vi "Log_ADAM_scan_table.vi"() -> ()   [LabVIEW 2010]
uses:
  ADAM Client/Sub VIs/ADAM Controls/Channel_State.ctl
  Anemometry/Anemometry Sub Vis/Globals/Constants_global.vi
  Anemometry/Anemometry Sub Vis/Globals/Preference_global.vi
  ADAM_Global.vi
  Anemometry/Anemometry Sub Vis/Globals/Meas_global.vi
panel:
  in  "Averaging time (Seconds)":dbl=60.0
  out "Current time":string
  out "Started Time":string
  in  "stop":bool
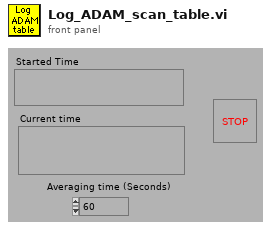
[diagram p1: front panel]
types:
  T1 = enum16{"On", "Off", "Always On", "Always Off", "Delete"}
  T2 = typedef "Channel_State.ctl" = enum16{"On", "Off", "Always On", "Always Off"}
  T3 = enum16{"Load ADAM setup from excel file", "Save ADAM setup to excel file"}
  T4 = cluster{"second":i32, "minute":i32, "hour":i32, "day of month":i32, "month":i32, "year":i32, "day of week":i32, "day of year":i32, "is DST":i32}
  T5 = typedef "Client_State_Cluster.ctl" = cluster{"Client Name":string, "Traverse level State":T6, "People to Email":string[], "Next Contact Time":dbl}
  T6 = typedef "Traverse_Level_State.ctl" = enum16{"Running", "Complete"}
  T7 = typedef "Server_Control.ctl" = cluster{"Channel Name to control":string, "Channel sharing":enum16{"Channel Unshared", "Channel Shared by Rig", "Channel Shared by Group"}, "Default Value":dbl, "Client Array":string[], "Time Stamp":timestamp, "Do Not Reset":bool}
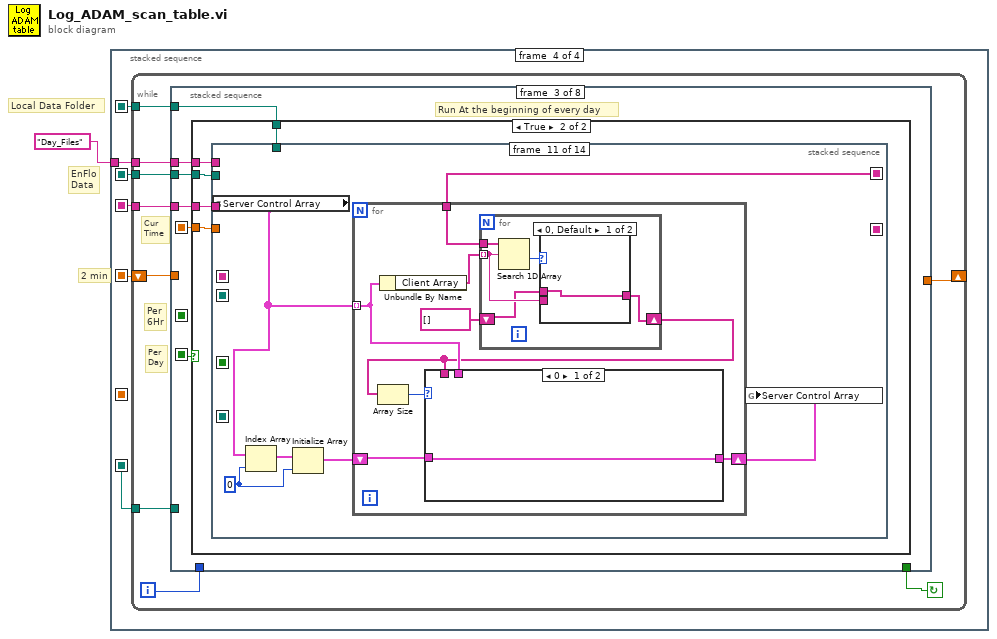
[diagram p0: block diagram]
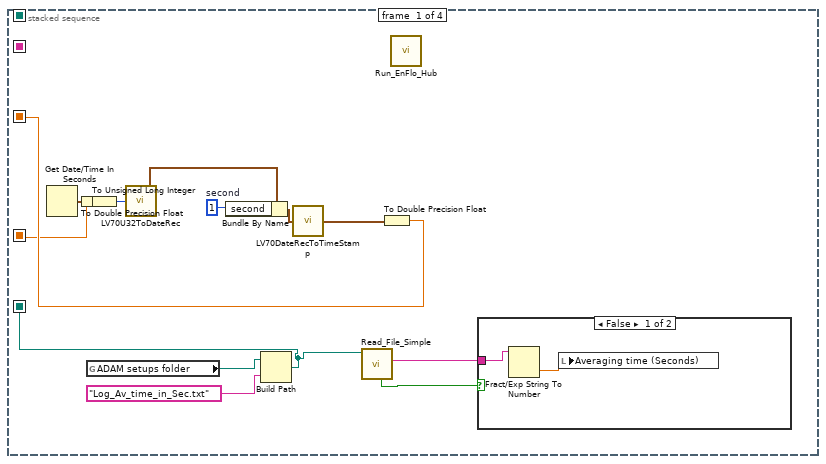
[diagram p2: hidden frame]
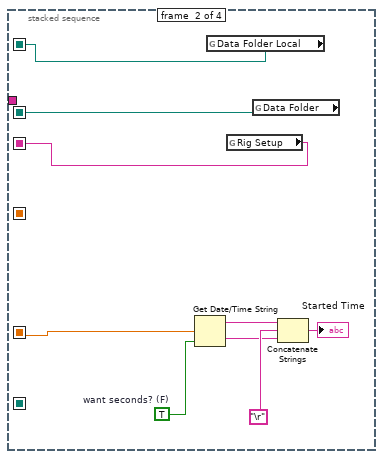
[diagram p4: hidden frame]
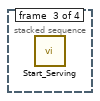
[diagram p5: hidden frame]
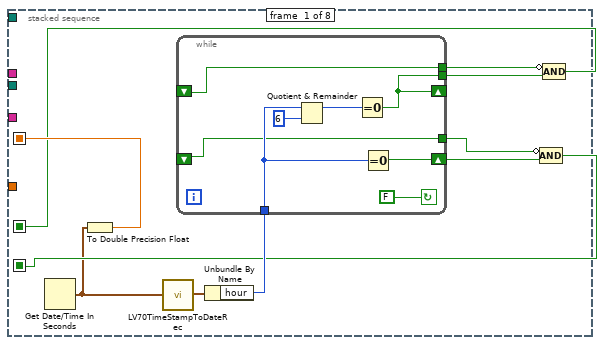
[diagram p6: hidden frame]
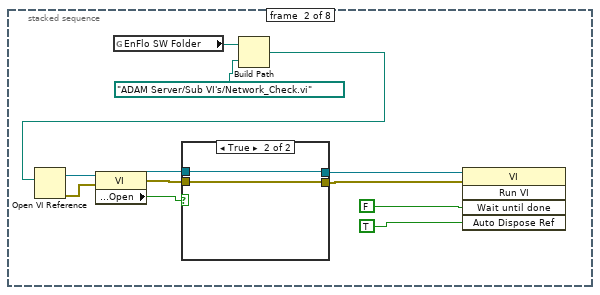
[diagram p7: hidden frame]
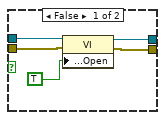
[diagram p8: hidden frame]
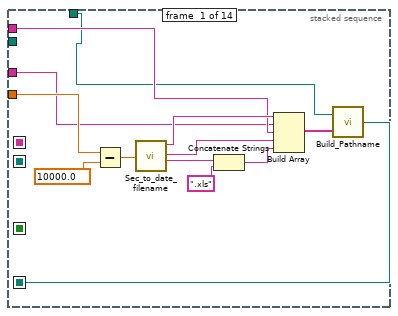
[diagram p10: hidden frame]
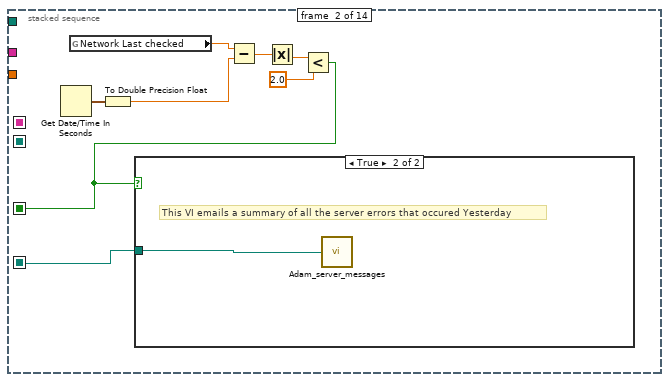
[diagram p11: hidden frame]
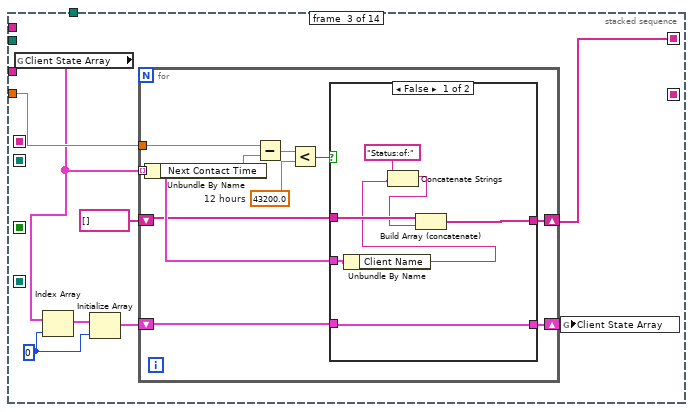
[diagram p13: hidden frame]
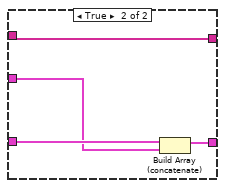
[diagram p14: hidden frame]
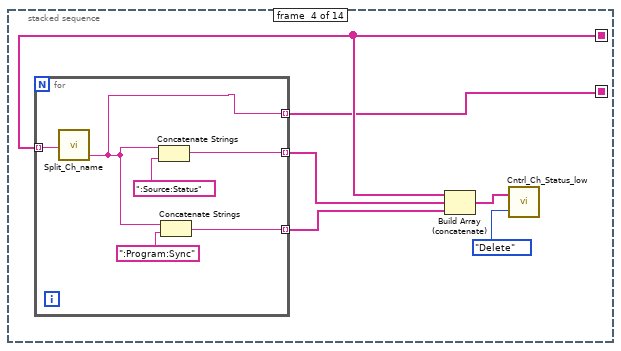
[diagram p15: hidden frame]
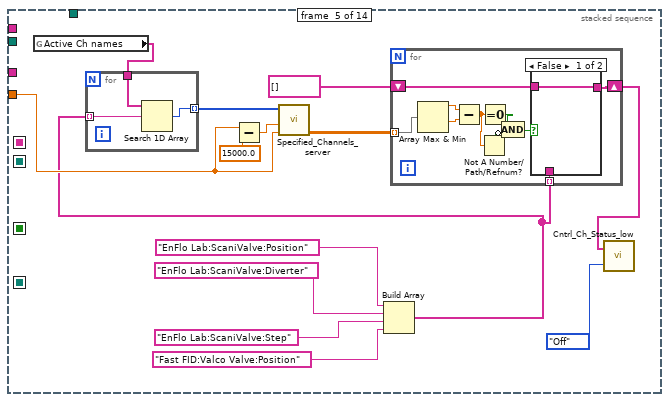
[diagram p16: hidden frame]
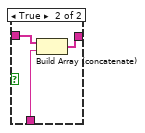
[diagram p17: hidden frame]
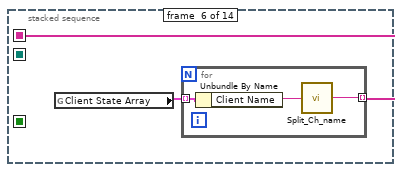
[diagram p18: hidden frame]
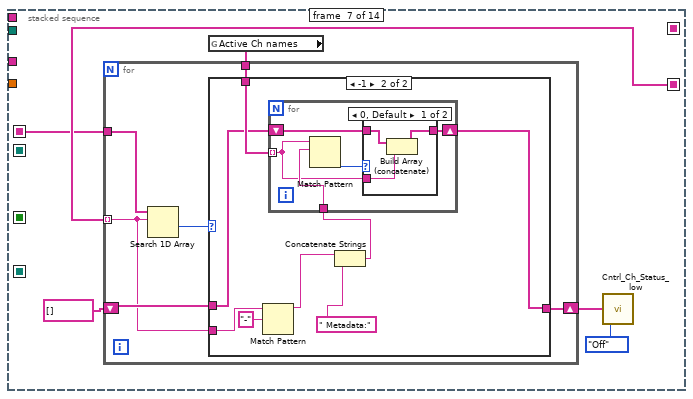
[diagram p19: hidden frame]
diagram:
  # "Local Data Folder"
  # "EnFlo\nData"
  # "2 min"
  n1 = stacked-sequence {
    seq-local: [w12 _ _ _] -> [_ _ _ w31]
    seq-local: [w11 _ _ _] -> [_ w25 _ _]
    seq-local: [_ w19 _ _] -> [_ _ _ w30]
    seq-local: [w4 _ _ _] -> [_ _ _ w28]
    seq-local: [_ w18 _ _] -> [_ _ _ w27]
    seq-local: [_ w17 _ _] -> [_ _ _ w26]
    tunnel: "Day_Files" ("Input Element") -> [_ _ _ w29]
    frame #0 {
      w14 = 1  # second
      n2 = Get Date/Time In Seconds() -> (seconds since 1Jan1904=w8:timestamp)
      n3 = To Double Precision Float(number=w8) -> (double precision float=w11:dbl)
      n4 = global read "Constants_global.vi" "ADAM setups folder"() -> (w6:path)
      n5 = To Unsigned Long Integer(number=w11) -> (unsigned 32bit integer=w10:u32)
      n6 = call <vilib>:"LV70U32ToDateRec.vi"("Time"=w10) -> ("date time rec"=w9:T4)
      n7 = Bundle By Name(cluster=w9, "second"=w14) -> (w13:T4)
      n8 = Build Path(base path=w6, name or relative path="Log_Av_time_in_Sec.txt") -> (appended path=w4:path)
      n9 = call <vilib>:"LV70DateRecToTimeStamp.vi"("date time rec"=w13) -> ("Time Stamp"=w7:timestamp)
      n10 = call "Read_File_Simple.vi"("Filename"=w4) -> ("Error?"=w2:bool, "string"=w3:string)  [unwired: 2 in, 6 out]
      n11 = To Double Precision Float(number=w7) -> (double precision float=w12:dbl)
      n12 = call "Run_EnFlo_Hub.vi"() -> ()  [unwired: 8 out]
      n13 = case shown="False" w2 {
        tunnel: w3 -> [w16 _]
        frame False {
          n14 = Fract/Exp String To Number(string=w16) -> (number=w15:dbl)  [unwired: 4 out]
          n15 = local write "Averaging time (Seconds)"(w15) -> ()
        }
        frame True {
        }
      }
    }
    frame #1 {
      w24 = TRUE  # want seconds? (F)
      n16 = Get Date/Time String(seconds (now)=w25, want seconds? (F)=w24) -> (date string=w22:string, time string=w21:string)  [unwired: 1 out]
      n17 = global read "Constants_global.vi" "Data Folder Local"() -> (w17:path)
      n18 = global read "Preference_global.vi" "Rig Setup"() -> (w18:string)
      n19 = global read "Constants_global.vi" "Data Folder"() -> (w19:path)
      n20 = Concatenate Strings(w22, "\r", w21) -> (→"Started Time":string)
    }
    frame #2 {
      n21 = call "Start_Serving.vi"() -> ()  [unwired: 1 out]
    }
    frame #3 {
      n22 = while {
        tunnel: w30 -> [w38]
        shift-left: w31 -> [w40]
        shift-right: [w39] -> _
        tunnel: w29 -> [w35]
        tunnel: w28 -> [w34]
        tunnel: w27 -> [w33]
        tunnel: w26 -> [w32]
        i -> [w37]
        stop <- w36 continue-if-true
        # "Per\n6Hr"
        # "Per\nDay"
        # "Cur\nTime"
        n23 = stacked-sequence {
          seq-local: [w42 _ _ _ _ _ _ _] -> [_ _ w83 _ _ _ _ _]
          seq-local: [w49 _ _ _ _ _ _ _] -> [_ _ w82 w342 _ w359 _ _]
          seq-local: [w45 _ _ _ _ _ _ _] -> [_ _ _ w336 _ _ _ _]
          tunnel: [_ _ _ _ _ w358 _ _] -> w39
          tunnel: w40 -> [_ _ _ _ _ w360 _ _]
          tunnel: w38 -> [_ _ w81 _ _ w367 _ _]
          tunnel: w37 -> [_ _ _ w335 _ _ _ _]
          tunnel: [_ _ _ _ _ _ _ w416] -> w36
          tunnel: w35 -> [_ _ w80 _ _ w368 _ _]
          tunnel: w34 -> [_ _ _ _ _ _ _ w415]
          tunnel: w33 -> [_ _ w79 _ _ w361 _ _]
          tunnel: w32 -> [_ _ w78 _ _ w357 _ _]
          frame #0 {
            n24 = Get Date/Time In Seconds() -> (seconds since 1Jan1904=w41:timestamp)
            n25 = To Double Precision Float(number=w41) -> (double precision float=w49:dbl)
            n26 = call <vilib>:"LV70TimeStampToDateRec.vi"("time stamp"=w41) -> ("date time rec"=w50:T4)
            n27 = Unbundle By Name(w50) -> ("hour"=w48:i32)
            n28 = while {
              tunnel: [w52] -> w43
              shift-left: _ -> [w52]
              shift-right: [w53] -> w44
              tunnel: [w55] -> w46
              tunnel: [w56] -> w47
              tunnel: w48 -> [w54]
              shift-left: _ -> [w55]
              shift-right: [w56] -> _
              stop <- FALSE continue-if-true
              n29 = Quotient & Remainder(x=w54, y=6) -> (x-y*floor(x/y)=w57:i32)  [unwired: 1 out]
              n30 = Equal To 0?(x=w57) -> (x = 0?=w56:bool)
              n31 = Equal To 0?(x=w54) -> (x = 0?=w53:bool)
            }
            n32 = Compound Arithmetic op=AND(invert w43, w44) -> (w42:bool)
            n33 = Compound Arithmetic op=AND(invert w46, w47) -> (w45:bool)
          }
          frame #1 {
            n34 = global read "Constants_global.vi" "EnFlo SW Folder"() -> (w68:path)
            n35 = Build Path(base path=w68, name or relative path=path "ADAM Server/Sub VI's/Network_Check.vi") -> (appended path=w69:path)
            n36 = Open VI Reference(vi path=w69) -> (vi reference=w65:refnum<vi>, error out=w64:errorcluster)  [unwired: 1 in, 4 out]
            n37 = property class="VI"(reference=w65, error in=w64) -> (reference out=w62:refnum<vi>, error out=w61:errorcluster, "Front Panel Window:Open"=w63:bool)
            n38 = case shown="True" w63 {
              tunnel: w62 -> [w74 w77]
              tunnel: w61 -> [w73 w76]
              tunnel: [w72 w77] -> w60
              tunnel: [w71 w76] -> w59
              frame False {
                n39 = property class="VI"(reference=w74, error in=w73, "Front Panel Window:Open"=TRUE) -> (reference out=w72:refnum<vi>, error out=w71:errorcluster)
              }
              frame True {
              }
            }
            n40 = invoke class="VI" method="Run VI"(reference=w60, error in=w59, "Wait until done"=FALSE, "Auto Dispose Ref"=TRUE) -> ()  [unwired: 1 in, 5 out]
          }
          frame #2 {
            # "Run At the beginning of every day"
            n41 = case shown="True" w83 {
              tunnel: w82 -> [_ w88]
              tunnel: w81 -> [_ w87]
              tunnel: w80 -> [_ w86]
              tunnel: w79 -> [_ w85]
              tunnel: w78 -> [_ w84]
              frame False {
              }
              frame True {
                n42 = stacked-sequence {
                  seq-local: [_ _ w111 _ _ _ _ _ _ _ _ _ _ _] -> [_ _ _ w145 _ _ _ _ _ _ w266 _ _ _]
                  seq-local: [w96 _ _ _ _ _ _ _ _ _ _ _ _ _] -> [_ w109 _ _ _ _ _ _ _ _ _ _ _ _]
                  seq-local: [_ _ _ w141 _ _ _ _ _ _ _ _ _ _] -> [_ _ _ _ _ _ w193 _ _ _ _ _ _ _]
                  seq-local: [_ _ _ _ _ w183 _ _ _ _ _ _ _ _] -> [_ _ _ _ _ _ w190 _ _ _ _ _ _ _]
                  seq-local: [_ _ _ _ _ _ _ _ _ _ _ _ w316 _] -> [_ _ _ _ _ _ _ _ _ _ _ _ _ w319]
                  seq-local: [_ w102 _ _ _ _ _ _ _ _ _ _ _ _] -> [_ _ _ _ _ _ _ _ w246 _ _ w294 _ w318]
                  tunnel: w88 -> [w100 _ w118 _ w162 _ _ _ _ _ _ w295 _ w320]
                  tunnel: w87 -> [_ _ _ _ _ _ _ _ _ _ _ _ _ _]
                  tunnel: w86 -> [w94 _ _ _ _ _ _ _ _ _ _ _ _ _]
                  tunnel: w85 -> [w90 _ _ _ _ _ _ _ _ _ _ _ _ _]
                  tunnel: w84 -> [w89 _ _ _ _ _ _ _ _ _ _ _ _ _]
                  frame #0 {
                    n43 = Subtract(x=w100, y=10000.0) -> (x-y=w98:dbl)
                    n44 = call "Sec_to_date_filename.vi"("seconds"=w98) -> ("Year"=w95:string, "Month"=w99:string, "Day"=w92:string)  [unwired: 1 out]
                    n45 = Concatenate Strings(w92, ".xls" ("string")) -> (w91:string)
                    n46 = Build Array(w95, w90, w94, w99, w91) -> (w97:string[])
                    n47 = call "Build_Pathname.vi"("Output Array"=w97, "Pathname"=w89) -> ("Appended path"=w96:path)
                  }
                  frame #1 {
                    n48 = Get Date/Time In Seconds() -> (seconds since 1Jan1904=w107:timestamp)
                    n49 = global read "ADAM_Global.vi" "Network Last checked"() -> (w104:dbl)
                    n50 = To Double Precision Float(number=w107) -> (double precision float=w108:dbl)
                    n51 = Subtract(x=w104, y=w108) -> (x-y=w105:dbl)
                    n52 = Absolute Value(x=w105) -> (abs(x)=w103:dbl)
                    n53 = Less?(x=w103, y=2.0) -> (x < y?=w102:bool)
                    n54 = case shown="True" w102 {
                      tunnel: w109 -> [_ w110]
                      frame False {
                      }
                      frame True {
                        # "This VI emails a summary of all the server errors that occured Yesterday"
                        n55 = call "Adam_server_messages.vi"("Filename"=w110) -> ()  [unwired: 1 out]
                      }
                    }
                  }
                  frame #2 {
                    w116 = 0 ("Index")
                    n56 = global read "ADAM_Global.vi" "Client State Array"() -> (w117:T5[])
                    n57 = Index Array(array=w117, index=w116) -> (element=w115:T5)
                    n58 = Initialize Array(w115, w116) -> (w114:T5[])
                    n59 = for {
                      tunnel: w117 -> [w121] mode=indexing
                      shift-right: [w122] -> w113
                      shift-left: w114 -> [w123]
                      tunnel: w118 -> [w128]
                      shift-right: [w119] -> w111
                      shift-left: string[] [] -> [w120]
                      w125 = 43200.0  # 12 hours
                      n60 = Unbundle By Name(w121) -> ("Next Contact Time"=w127:dbl)
                      n61 = Subtract(x=w128, y=w127) -> (x-y=w126:dbl)
                      n62 = Less?(x=w126, y=w125) -> (x < y?=w124:bool)
                      n63 = case shown="False" w124 {
                        tunnel: w123 -> [w135 w139]
                        tunnel: [w135 w138] -> w122
                        tunnel: w121 -> [w134 w137]
                        tunnel: w120 -> [w133 w136]
                        tunnel: [w132 w136] -> w119
                        frame False {
                          n64 = Unbundle By Name(w134) -> ("Client Name"=w130:string)
                          n65 = Concatenate Strings("Status:of:", w130) -> (w129:string)
                          n66 = Build Array (concatenate)(w133, w129) -> (w132:string[])
                        }
                        frame True {
                          n67 = Build Array (concatenate)(w139, w137) -> (w138:T5[])
                        }
                      }
                    }
                    n68 = global write "ADAM_Global.vi" "Client State Array"(w113) -> ()
                  }
                  frame #3 {
                    n69 = for {
                      tunnel: w145 -> [w151] mode=indexing
                      tunnel: [w148] -> w143 mode=indexing
                      tunnel: [w147] -> w142 mode=indexing
                      tunnel: [w146] -> w141 mode=indexing
                      n70 = call "Split_Ch_name.vi"("Ch name"=w151) -> ("Low level"=w146:string)  [unwired: 2 out]
                      n71 = Concatenate Strings(w146, ":Source:Status") -> (w148:string)
                      n72 = Concatenate Strings(w146, ":Program:Sync") -> (w147:string)
                    }
                    n73 = Build Array (concatenate)(w145, w143, w142) -> (w144:string[])
                    n74 = call "Cntrl_Ch_Status_low.vi"("Mode"=T1."Delete", "Channel names"=w144) -> ()  [unwired: 1 out]
                  }
                  frame #4 {
                    n75 = global read "ADAM_Global.vi" "Active Ch names"() -> (w165:string[])
                    n76 = Subtract(x=w162, y=15000.0) -> (x-y=w160:dbl)
                    n77 = Build Array("EnFlo Lab:ScaniValve:Position", "EnFlo Lab:ScaniValve:Diverter", "EnFlo Lab:ScaniValve:Step", "Fast FID:Valco Valve:Position") -> (w158:string[])
                    n78 = for {
                      tunnel: w165 -> [w182]
                      tunnel: w158 -> [w181] mode=indexing
                      tunnel: [w180] -> w163 mode=indexing
                      n79 = Search 1D Array(1D array=w182, element=w181) -> (index of element=w180:i32)  [unwired: 1 out]
                    }
                    n80 = call "Specified_Channels_server.vi"("End time"=w162, "Start time"=w160, "Requested channels"=w163) -> ("Output array"=w159:dbl[][])  [unwired: 2 in, 4 out]
                    n81 = for {
                      tunnel: w159 -> [w172] mode=indexing
                      shift-right: [w173] -> w153
                      shift-left: string[] [] -> [w167]
                      tunnel: w158 -> [w168] mode=indexing
                      n82 = Array Max & Min(array=w172) -> (max value=w175:dbl, min value=w174:dbl)  [unwired: 2 out]
                      n83 = Subtract(x=w175, y=w174) -> (x-y=w171:dbl)
                      n84 = Not A Number/Path/Refnum?(number/path/refnum=w171) -> (NaN/Path/Refnum?=w169:bool)
                      n85 = Equal To 0?(x=w171) -> (x = 0?=w166:bool)
                      n86 = Compound Arithmetic op=AND(w166, invert w169) -> (w170:bool)
                      n87 = case shown="False" w170 {
                        tunnel: [w176 w179] -> w173
                        tunnel: w168 -> [_ w178]
                        tunnel: w167 -> [w176 w177]
                        frame False {
                        }
                        frame True {
                          n88 = Build Array (concatenate)(w177, w178) -> (w179:string[])
                        }
                      }
                    }
                    n89 = call "Cntrl_Ch_Status_low.vi"("Mode"=T1."Off", "Channel names"=w153) -> ()  [unwired: 1 out]
                  }
                  frame #5 {
                    n90 = global read "ADAM_Global.vi" "Client State Array"() -> (w184:T5[])
                    n91 = for {
                      tunnel: w184 -> [w187] mode=indexing
                      tunnel: [w185] -> w183 mode=indexing
                      n92 = Unbundle By Name(w187) -> ("Client Name"=w186:string)
                      n93 = call "Split_Ch_name.vi"("Ch name"=w186) -> ("Middle"=w185:string)  [unwired: 2 out]
                    }
                  }
                  frame #6 {
                    n94 = global read "ADAM_Global.vi" "Active Ch names"() -> (w191:string[])
                    n95 = for {
                      tunnel: w193 -> [w194] mode=indexing
                      shift-right: [w197] -> w189
                      shift-left: string[] [] -> [w198]
                      tunnel: w191 -> [w196]
                      tunnel: w190 -> [w195]
                      n96 = Search 1D Array(1D array=w195, element=w194) -> (index of element=w199:i32)  [unwired: 1 out]
                      n97 = case shown="-1" w199 {
                        tunnel: w198 -> [w200 w206]
                        tunnel: [w200 w205] -> w197
                        tunnel: w194 -> [_ w201]
                        tunnel: w196 -> [_ w207]
                        frame 0, Default {
                        }
                        frame -1 {
                          n98 = Match Pattern(string=w201, regular expression="-") -> (before substring=w202:string)  [unwired: 4 out]
                          n99 = Concatenate Strings(w202, " Metadata:" ("Substring")) -> (w204:string)
                          n100 = for {
                            shift-right: [w211] -> w205
                            shift-left: w206 -> [w212]
                            tunnel: w204 -> [w210]
                            tunnel: w207 -> [w209] mode=indexing
                            n101 = Match Pattern(string=w209, regular expression=w210) -> (offset past match=w213:i32)  [unwired: 4 out]
                            n102 = case shown="0, Default" w213 {
                              tunnel: w212 -> [w215 w217]
                              tunnel: [w214 w217] -> w211
                              tunnel: w209 -> [w216 _]
                              frame 0, Default {
                                n103 = Build Array (concatenate)(w215, w216) -> (w214:string[])
                              }
                              frame -1 {
                              }
                            }
                          }
                        }
                      }
                    }
                    n104 = call "Cntrl_Ch_Status_low.vi"("Mode"=T1."Off", "Channel names"=w189) -> ()  [unwired: 1 out]
                  }
                  frame #7 {
                    n105 = Build Array("EnFlo_Tunnel:Heater:Enable") -> (w223:string[])
                    n106 = call "Get_Current_Scan_server.vi"("Desired Channels"=w223) -> ("Numerical Values"=w222:dbl[])  [unwired: 2 out]
                    n107 = Index Array(array=w222, index=0) -> (element=w220:dbl)
                    n108 = Less?(x=w220, y=0.5) -> (x < y?=w218:bool)
                    n109 = case shown="True" w218 {
                      frame False {
                      }
                      frame True {
                        w229 = "EnFlo_Tunnel:Setpo"
                        n110 = global read "ADAM_Global.vi" "Active Ch names"() -> (w227:string[])
                        n111 = String Length(string=w229) -> (length=w228:i32)
                        n112 = for {
                          shift-right: [w237] -> w226
                          shift-left: string[] [] -> [w239]
                          tunnel: w227 -> [w238] mode=indexing
                          tunnel: w228 -> [w241]
                          tunnel: w229 -> [w240]
                          tunnel: "EnFlo_Tunnel:Power" -> [w235]
                          n113 = String Subset(string=w238, length (rest)=w241) -> (substring=w236:string)  [unwired: 1 out]
                          n114 = Equal?(x=w236, y=w240) -> (x = y?=w233:bool)
                          n115 = Equal?(x=w236, y=w235) -> (x = y?=w234:bool)
                          n116 = Or(x=w233, y=w234) -> (x .or. y?=w232:bool)
                          n117 = case shown="True" w232 {
                            tunnel: w239 -> [w242 w245]
                            tunnel: w238 -> [_ w244]
                            tunnel: [w242 w243] -> w237
                            frame False {
                            }
                            frame True {
                              n118 = Build Array (concatenate)(w245, w244) -> (w243:string[])
                            }
                          }
                        }
                        n119 = call "Adam_Ch_on_off.vi"("Ch State"=Channel_State."Off", "ADAM Ch Names"=w226) -> ()  [unwired: 1 out]
                      }
                    }
                  }
                  frame #8 {
                    n120 = case shown="True" w246 {
                      frame False {
                      }
                      frame True {
                        n121 = call "Read_Write_ADAM_setup.vi"("Mode"=T3."Save ADAM setup to excel file") -> ()  [unwired: 4 out]
                      }
                    }
                  }
                  frame #9 {
                    w251 = 5400.0  # 1.5 Hrs in seconds
                    n122 = Build Array("GMU:Source:Meas Q", "GMU:Source:Est Time") -> (w258:string[])
                    n123 = call "Get_Current_Scan_server.vi"("Desired Channels"=w258) -> ("Numerical Values"=w253:dbl[])  [unwired: 2 out]
                    n124 = Index Array(array=w253, index=0 ("Index")) -> (element=w255:dbl)
                    n125 = Index Array(array=w253, index=1 ("Index")) -> (element=w252:dbl)
                    n126 = Less?(x=w255, y=0.01) -> (x < y?=w249:bool)
                    n127 = Greater?(x=w252, y=w251) -> (0:w250:bool)
                    n128 = And(x=w249, y=w250) -> (x .and. y?=w248:bool)
                    n129 = case shown="True" w248 {
                      frame False {
                      }
                      frame True {
                        w261 = FALSE  # Activate channels
                        w262 = enum16{"Channel Name", "Main Address"}."Channel Name" ("Control on")
                        n130 = call "Ch_Active_Control.vi"("Match"="GMU:", "Activate Channels?"=w261, "Control on"=w262) -> ()  [unwired: 1 in, 2 out]
                        n131 = call "Ch_Active_Control.vi"("Match"="source", "Activate Channels?"=w261, "Control on"=w262) -> ()  [unwired: 1 in, 2 out]
                      }
                    }
                  }
                  frame #10 {
                    w270 = 0 ("Index")
                    n132 = global read "ADAM_Global.vi" "Server Control Array"() -> (w267:T7[])
                    n133 = Index Array(array=w267, index=w270) -> (element=w269:T7)
                    n134 = Initialize Array(w269, w270) -> (w268:T7[])
                    n135 = for {
                      tunnel: w267 -> [w272] mode=indexing
                      shift-right: [w277] -> w265
                      shift-left: w268 -> [w278]
                      tunnel: w266 -> [w276]
                      n136 = Unbundle By Name(w272) -> ("Client Array"=w275:string[])
                      n137 = for {
                        tunnel: w276 -> [w283]
                        tunnel: w275 -> [w281] mode=indexing
                        shift-right: [w279] -> w271
                        shift-left: string[] [] -> [w280]
                        n138 = Search 1D Array(1D array=w283, element=w281) -> (index of element=w282:i32)  [unwired: 1 out]
                        n139 = case shown="0, Default" w282 {
                          tunnel: w281 -> [_ w287]
                          tunnel: w280 -> [w284 w286]
                          tunnel: [w284 w285] -> w279
                          frame 0, Default {
                          }
                          frame -1 {
                            n140 = Build Array (concatenate)(w286, w287) -> (w285:string[])
                          }
                        }
                      }
                      n141 = Array Size(array=w271) -> (size(s)=w273:i32)
                      n142 = case shown="0" w273 {
                        tunnel: w278 -> [w288 w292]
                        tunnel: [w288 w293] -> w277
                        tunnel: w272 -> [_ w291]
                        tunnel: w271 -> [_ w290]
                        frame 0 {
                        }
                        frame 1, Default {
                          n143 = Bundle By Name(cluster=w291, "Client Array"=w290) -> (w289:T7)
                          n144 = Build Array (concatenate)(w292, w289) -> (w293:T7[])
                        }
                      }
                    }
                    n145 = global write "ADAM_Global.vi" "Server Control Array"(w265) -> ()
                  }
                  frame #11 {
                    n146 = case shown="True" w294 {
                      frame False {
                      }
                      frame True {
                        w303 = "\r"
                        n147 = global read "Constants_global.vi" "ADAM setups folder"() -> (w306:path)
                        n148 = Build Path(base path=w306, name or relative path="Setup_Files") -> (appended path=w310:path)
                        n149 = Build Path(base path=w306, name or relative path="Hi_Tec_Calibs.xls") -> (appended path=w305:path)
                        n150 = Build Path(base path=w310, name or relative path="Selected_Filename.txt" ("Substring")) -> (appended path=w312:path)
                        n151 = call "Read_File_Simple.vi"("Filename"=w312) -> ("string"=w311:string)  [unwired: 2 in, 7 out]
                        n152 = Build Path(base path=w310, name or relative path=w311) -> (appended path=w309:path)
                        n153 = call "Read_File_Simple.vi"("Filename"=w305) -> ("string"=w304:string)  [unwired: 2 in, 7 out]
                        n154 = call "Read_File_Simple.vi"("Filename"=w309) -> ("string"=w308:string)  [unwired: 2 in, 7 out]
                        n155 = call "Get_mod_dates.vi"() -> ("Output string"=w302:string)  [unwired: 1 in, 4 out]
                        n156 = call "Create_Error_log_folders.vi"("Per Day Log File?"=TRUE, "Log Filename"="ADAM_Setups" ("Substring")) -> ("Server copy Location"=w296:path, "Local Log File"=w298:path)  [unwired: 1 in, 1 out]
                        n157 = Concatenate Strings(w308, w303, w304, w303, w302) -> (w299:string)
                        n158 = call "Write_File_Simple.vi"("character string"=w299, "file path"=w298) -> ("file path Out"=w297:path)  [unwired: 1 in, 1 out]
                        n159 = call "Updated_File_Copy.vi"("Target Path"=w296, "Source Path"=w297) -> ()  [unwired: 2 out]
                      }
                    }
                    n160 = global write "Meas_global.vi" "Start Time of experiment"(w295) -> ()
                  }
                  frame #12 {
                    n161 = global read "Constants_global.vi" "Data Folder Local"() -> (w317:path)
                    n162 = Build Path(base path=w317, name or relative path="Results_Summary_files") -> (appended path=w316:path)
                  }
                  frame #13 {
                    n163 = case shown="True" w318 {
                      tunnel: w320 -> [_ w323]
                      tunnel: w319 -> [_ w321]
                      frame False {
                      }
                      frame True {
                        # "If the summary files are more than 60 days old delete them"
                        n164 = To Unsigned Long Integer(number=w323) -> (unsigned 32bit integer=w322:u32)
                        n165 = call "Get_folder_and_filenames.vi"("file path (dialog if empty)"=w321) -> ("Files"=w324:path[])  [unwired: 1 out]
                        n166 = for {
                          tunnel: w324 -> [w326] mode=indexing
                          tunnel: w322 -> [w331]
                          # "60 days in seconds"
                          n167 = File/Directory Info(path=w326) -> (last mod=w325:timestamp)  [unwired: 1 in, 6 out]
                          n168 = To Unsigned Long Integer(number=w325) -> (unsigned 32bit integer=w330:u32)
                          n169 = Subtract(x=w331, y=w330) -> (x-y=w329:u32)
                          n170 = Greater?(x=w329, y=u32 5184000) -> (0:w327:bool)
                          n171 = case shown="True" w327 {
                            tunnel: w326 -> [_ w332]
                            frame False {
                            }
                            frame True {
                              n172 = Delete(path (use dialog)=w332) -> ()  [unwired: 1 in, 6 out]
                            }
                          }
                        }
                      }
                    }
                  }
                }
              }
            }
          }
          frame #3 {
            n173 = global read "ADAM_Global.vi" "Network Last checked"() -> (w341:dbl)
            n174 = Subtract(x=w342, y=w341) -> (x-y=w337:dbl)
            n175 = Greater?(x=w335, y=30) -> (0:w333:bool)
            n176 = Greater?(x=w337, y=25.0) -> (0:w339:bool)
            n177 = Compound Arithmetic op=AND(w339, w336, w333) -> (w338:bool)
            n178 = case shown="True" w338 {
              tunnel: w337 -> [_ w347]
              tunnel: w336 -> [w343 _]
              frame False {
                n179 = case shown="True" w343 {
                  frame False {
                  }
                  frame True {
                    n180 = call "Organise_Movies.vi"() -> ()  [unwired: 1 out]
                  }
                }
              }
              frame True {
                n181 = Divide(x=w347, y=60.0) -> (x/y=w345:dbl)
                n182 = global read "Constants_global.vi" "ADAM setups folder"() -> (w355:path)
                n183 = Path to Array of Strings(0:w355) -> (2:w349:string[])  [unwired: 1 out]
                n184 = Index Array(array=w349, index=0) -> (element=w351:string)
                n185 = Format Into String(format string="%s Offline", w351) -> (resulting string=w353:string)  [unwired: 2 in, 1 out]
                n186 = Format Into String(format string="The file %s has been Offline now for %d minutes", w355, w345) -> (resulting string=w344:string)  [unwired: 2 in, 1 out]
                n187 = call "Server_Emails.vi"("Message"=w344, "Contact All clients?"=TRUE, "Subject"=w353) -> ()  [unwired: 2 in, 3 out]
              }
            }
          }
          frame #4 {
            n188 = Wait (ms)(milliseconds to wait=u32 1000 ("milliseconds to Wait")) -> ()  [unwired: 1 out]
          }
          frame #5 {
            n189 = Divide(x="Averaging time (Seconds)", y=60.0) -> (x/y=w365:dbl)
            n190 = Divide(x="Averaging time (Seconds)", y=2.0) -> (x/y=w362:dbl)
            n191 = Add(x=w362, y=w360) -> (x+y=w378:dbl)
            n192 = call "Sec_to_date_filename.vi"("seconds"=w378) -> ("Year"=w373:string, "Month"=w374:string, "Day"=w369:string)  [unwired: 1 out]
            n193 = Concatenate Strings(w369, ".xls" ("string")) -> (w371:string)
            n194 = Build Array(w373, w361, w368, w374, w371) -> (w372:string[])
            n195 = call "Time_elapsed.vi"("End of previous average in"=w360, "Averaging time (mins)"=w365) -> ("End of previous average out"=w358:dbl, "End of period"=w376:dbl, "Start of period"=w377:dbl, "Time elapsed ?"=w375:bool)  [unwired: 2 in]
            n196 = case shown="True" w375 {
              tunnel: w376 -> [_ w383]
              tunnel: w377 -> [_ w384]
              tunnel: w367 -> [_ w382]
              tunnel: w372 -> [_ w381]
              tunnel: w357 -> [_ w380]
              tunnel: w359 -> [_ w379]
              frame False {
              }
              frame True {
                n197 = stacked-sequence {
                  seq-local: [w385 _ _] -> [_ _ w404]
                  seq-local: [w387 _ _] -> [_ _ w406]
                  tunnel: w384 -> [w401 _ _]
                  tunnel: w383 -> [w400 _ _]
                  tunnel: w382 -> [_ _ w405]
                  tunnel: w381 -> [w396 _ w407]
                  tunnel: w380 -> [w395 _ _]
                  tunnel: w379 -> [w393 _ _]
                  frame #0 {
                    n198 = global read "ADAM_Global.vi" "Network Last checked"() -> (w394:dbl)
                    n199 = global read "ADAM_Global.vi" "2 Min average comment"() -> (w399:string)
                    n200 = global read "Meas_global.vi" "Error Messages"() -> (w398:string)
                    n201 = call "Build_Pathname.vi"("Output Array"=w396, "Pathname"=w395) -> ("Appended path"=w386:path)
                    n202 = call "Create_directory_path.vi"("Path name"=w386) -> ("Path name Out"=w385:path)
                    n203 = Subtract(x=w394, y=w393) -> (x-y=w392:dbl)
                    n204 = Concatenate Strings(w399, w398) -> (w397:string)
                    n205 = call "Write_to_log_file.vi"("User added comment"=w397, "End time"=w400, "Start time"=w401, "Folder/file"=w385) -> ("File Updated?"=w389:bool)  [unwired: 5 in, 2 out]
                    n206 = Absolute Value(x=w392) -> (abs(x)=w391:dbl)
                    n207 = Less?(x=w391, y=1.5) -> (x < y?=w388:bool)
                    n208 = And(x=w389, y=w388) -> (x .and. y?=w387:bool)
                  }
                  frame #1 {
                    w402 = ""
                    n209 = global write "ADAM_Global.vi" "2 Min average comment"(w402) -> ()
                    n210 = global write "Meas_global.vi" "Error Messages"(w402) -> ()
                  }
                  frame #2 {
                    n211 = call "Build_Pathname.vi"("Output Array"=w407, "Pathname"=w405) -> ("Appended path"=w403:path)
                    n212 = case shown="True" w406 {
                      tunnel: w404 -> [_ w409]
                      tunnel: w403 -> [_ w408]
                      frame False {
                      }
                      frame True {
                        n213 = call "Updated_File_Copy.vi"("Target Path"=w408, "Source Path"=w409) -> ()  [unwired: 2 out]
                      }
                    }
                  }
                }
              }
            }
          }
          frame #6 {
            w414 = TRUE  # want seconds? (F)
            n214 = Get Date/Time String(want seconds? (F)=w414) -> (date string=w412:string, time string=w411:string)  [unwired: 2 out]
            n215 = Concatenate Strings(w412, "\r", w411) -> (→"Current time":string)
          }
          frame #7 {
            n216 = while {
              shift-right: [w418] -> _
              shift-left: _ -> [w422]
              tunnel: w415 -> [w419]
              stop <- TRUE stop-if-true
              n217 = local read "Averaging time (Seconds)"() -> (w418:dbl)
              n218 = Not Equal?(x=w418, y=w422) -> (x != y?=w420:bool)
              n219 = case shown="True" w420 {
                tunnel: w419 -> [_ w423]
                tunnel: w418 -> [_ w425]
                frame False {
                }
                frame True {
                  n220 = Number To Fractional String(number=w425, precision (6)=i16 6) -> (F-format string=w424:string)  [unwired: 2 out]
                  n221 = call "Write_File_Simple.vi"("character string"=w424, "file path"=w423) -> ()  [unwired: 1 in, 2 out]
                }
              }
            }
            n222 = Not(x="stop") -> (.not. x?=w416:bool)
          }
        }
      }
    }
  }
